vi "Auto Scan Z move XY Sensitivity.vi"() -> ()   [LabVIEW 2014]
uses:
  Main-Stage-PI/(Global) Current handle and LaserPower_YCC.vi
panel:
  in  "# of Steps":i32=10
  in  "T=Z to up\nF=Z to down":bool
  in  "Z stepsize (nm)":dbl=20.0
  in  "Axis (XYZ)":enum16{"x", "y", "z"}(ring)
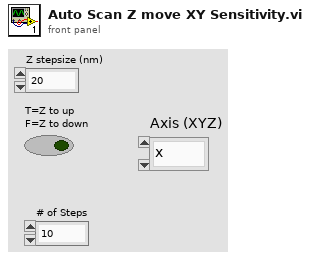
[diagram p1: front panel]
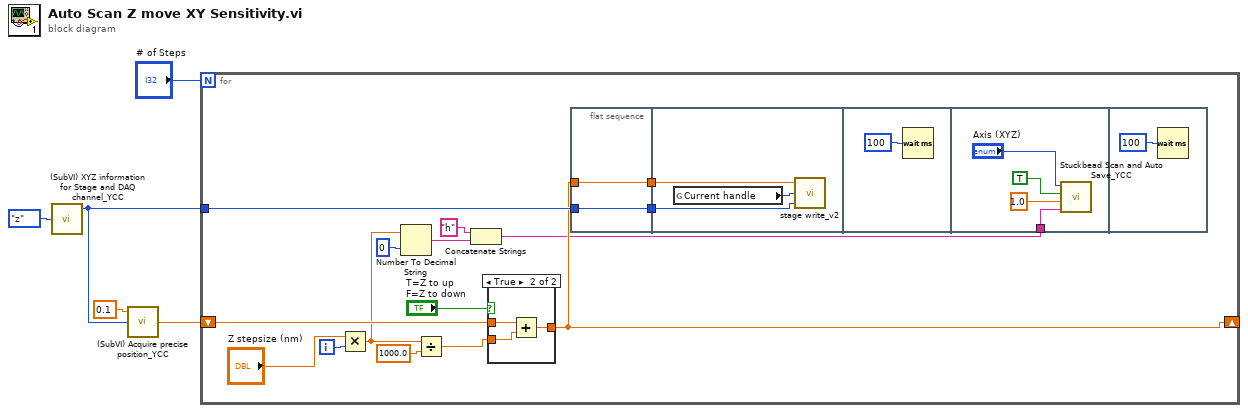
[diagram p0: block diagram]
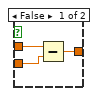
[diagram p2: hidden frame]
diagram:
  n1 = call "(SubVI) XYZ information for Stage and DAQ channel_YCC.vi"("Axis  (Enum)"=enum16{"x", "y", "z"}."z") -> ("Axis"=w3:i32)  [unwired: 3 in, 1 out]
  n2 = call "(SubVI) Acquire precise position_YCC.vi"("Axis"=w3, "record time (s)"=0.1) -> ("precise current position (um)"=w2:dbl)  [unwired: 3 in]
  n3 = for {
    N: "# of Steps" -> [_]
    tunnel: w3 -> [w20]
    shift-right: [w13] -> _
    shift-left: w2 -> [w15]
    i -> [w19]
    n4 = Multiply(x="Z stepsize (nm)", y=w19) -> (x*y=w11:dbl)
    n5 = Number To Decimal String(number=w11, width (-)=i16 0) -> (decimal integer string=w9:string)
    n6 = Divide(x=w11, y=1000.0) -> (x/y=w14:dbl)
    n7 = Concatenate Strings("h" ("string"), w9) -> (w8:string)
    n8 = case shown="True" "T=Z to up\nF=Z to down" {
      tunnel: w15 -> [w23 w26]
      tunnel: w14 -> [w22 w25]
      tunnel: [w21 w24] -> w13
      frame False {
        n9 = Subtract(x=w23, y=w22) -> (x-y=w21:dbl)
      }
      frame True {
        n10 = Add(x=w26, y=w25) -> (x+y=w24:dbl)
      }
    }
    n11 = flat-sequence {
      tunnel: w13 -> [w27]
      tunnel: w20 -> [w28]
      tunnel: [w28] -> w7
      tunnel: [w27] -> w6
      tunnel: w7 -> [w30]
      tunnel: w6 -> [w29]
      tunnel: w8 -> [w34]
      frame #0 {
      }
      frame #1 {
        n12 = global read "(Global) Current handle and LaserPower_YCC.vi" "Current handle"() -> (w31:i32)
        n13 = call "stage write_v2.vi"("axis"=w30, "Incoming Handle"=w31, "position"=w29) -> ()  [unwired: 2 in, 1 out]
      }
      frame #2 {
        n14 = Wait (ms)(milliseconds to wait=u32 100) -> ()  [unwired: 1 out]
      }
      frame #3 {
        n15 = call "Stuckbead Scan and Auto Save_YCC.vi"("File name add to the end"=w34, "Scan Range  (um)"=1.0, "Save Data?"=TRUE, "Axis (XYZ)"="Axis (XYZ)") -> ()  [unwired: 8 in]
      }
      frame #4 {
        n16 = Wait (ms)(milliseconds to wait=u32 100) -> ()  [unwired: 1 out]
      }
    }
  }
